vi "WB_add_sav_to_temp_WB_sub.vi"(0 "weigths_2D":dbl[][](array[numeric]), 1 "Export_weights_cvs":path=path "C:/Users/HYPC/Desktop/MNIST_pattern_Recognition Program/temp/temp_W.csv", 2 "biases_1d":dbl[](array[numeric]), 3 "format (%.3f)":string="%.3f", 4 "Export_biases_cvs":path=path "C:/Users/HYPC/Desktop/MNIST_pattern_Recognition Program/temp/temp_B.csv") -> (5 "Weights_2D_N":dbl[][](array[numeric]), 6 "biases_1d_N":dbl[](array[numeric]))   [LabVIEW 2021]
uses:
  <vilib>/Utility/file.llb/Read Delimited Spreadsheet (DBL).vi
  <vilib>/Utility/file.llb/Write Delimited Spreadsheet (DBL).vi
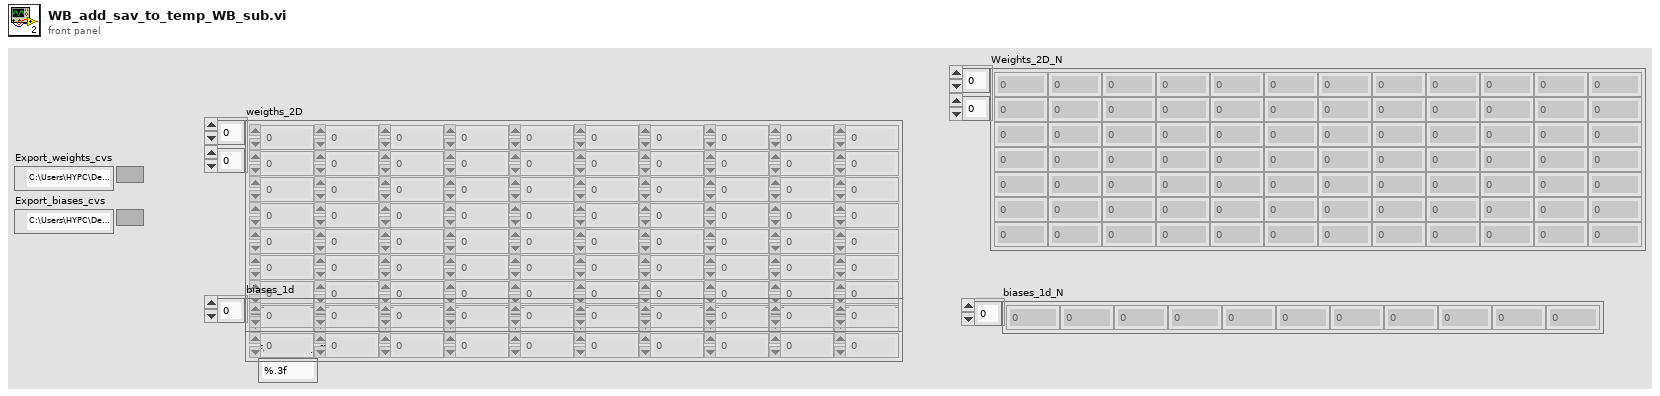
[diagram p1: front panel]
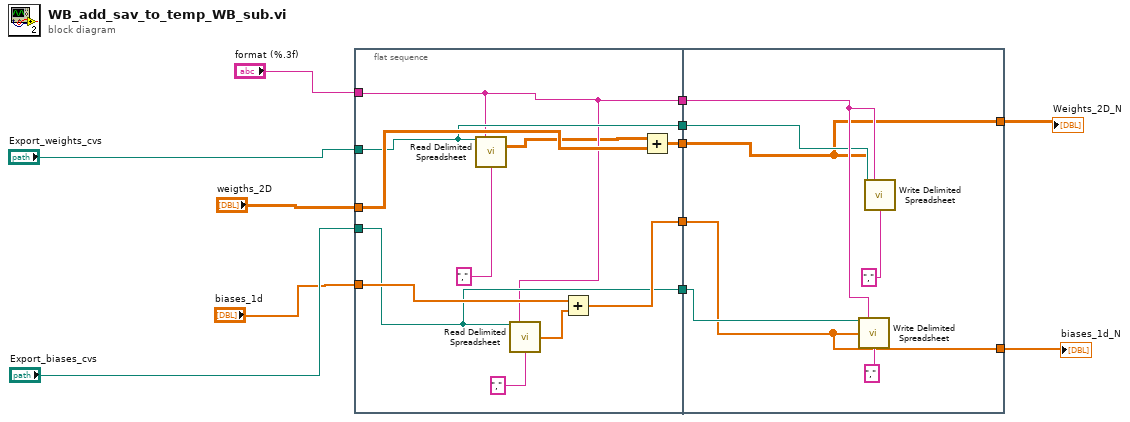
[diagram p0: block diagram]
diagram:
  n1 = flat-sequence {
    tunnel: "Export_weights_cvs" -> [w16]
    tunnel: "Export_biases_cvs" -> [w15]
    tunnel: "weigths_2D" -> [w19]
    tunnel: "biases_1d" -> [w20]
    tunnel: [w18] -> w12
    tunnel: [w17] -> w11
    tunnel: [w16] -> w10
    tunnel: [w15] -> w9
    tunnel: [w14] -> w8
    tunnel: "format (%.3f)" -> [w14]
    tunnel: w12 -> [w25]
    tunnel: w11 -> [w24]
    tunnel: w10 -> [w27]
    tunnel: w9 -> [w26]
    tunnel: w8 -> [w28]
    tunnel: [w25] -> w1
    tunnel: [w24] -> w3
    frame #0 {
      n2 = call-poly <vilib>:"Read Delimited Spreadsheet.vi"("file path (dialog if empty)"=w16, "format (%.3f)"=w14, "delimiter (\\t)"="," ("delimiter (\\t)")) -> ("all rows"=w13:dbl[][])  [unwired: 7 in, 5 out]
      n3 = call-poly <vilib>:"Read Delimited Spreadsheet.vi"("file path (dialog if empty)"=w15, "format (%.3f)"=w14, "delimiter (\\t)"="," ("delimiter (\\t)")) -> ("first row"=w21:dbl[])  [unwired: 7 in, 5 out]
      n4 = Add(x=w20, y=w21) -> (x+y=w17:dbl[])
      n5 = Add(x=w13, y=w19) -> (x+y=w18:dbl[][])
    }
    frame #1 {
      n6 = call-poly <vilib>:"Write Delimited Spreadsheet.vi"("file path (dialog if empty)"=w26, "format (%.3f)"=w28, "1D data"=w24, "delimiter (\\t)"="," ("delimiter (\\t)")) -> ()  [unwired: 10 in, 2 out]
      n7 = call-poly <vilib>:"Write Delimited Spreadsheet.vi"("file path (dialog if empty)"=w27, "format (%.3f)"=w28, "2D data"=w25, "delimiter (\\t)"="," ("delimiter (\\t)")) -> ()  [unwired: 10 in, 2 out]
    }
  }
  "Weights_2D_N" <- w1
  "biases_1d_N" <- w3
